vi "test - Convert config array - I8 - 1.vi"(8 "error in (no error)":errorcluster, 11 "TestCase in":refnum<class "Create New Assert Tester.lvclass">) -> (0 "error out":errorcluster, 3 "TestCase out":refnum<class "Create New Assert Tester.lvclass">)   [LabVIEW 2016, in "Create New Assert Tester.lvclass"]
uses:
  Create New Assert Tester.lvclass
  Plugins/Utility/Assert Build Configuration.ctl
  Core/Assert API Components/Failure Actions.ctl
  <vilib>/Utility/Data Type/Type Definitions/Data Type.ctl
  Plugins/Utility/Assert Scripting Configuration.ctl
  <vilib>/addons/_JKI Toolkits/VI Tester/TestCase.llb/TestCase.lvclass
  <vilib>/Utility/Data Type/NI_Data Type.lvlib
  Core/Assert API Components/Assert API Components.lvlib
  C:/Program Files (x86)/National Instruments/LabVIEW 2016/vi.lib/addons/_JKI Toolkits/VI Tester/TestCase.llb/TestCase.lvclass
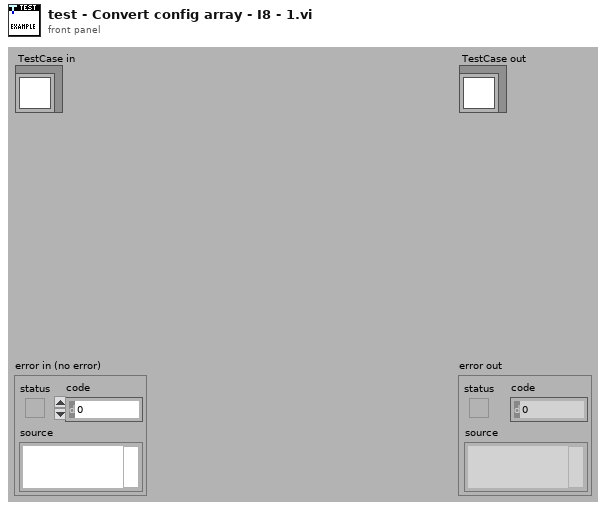
[diagram p1: front panel]
types:
  T1 = typedef "Assert Build Configuration.ctl" = cluster{"Assert Name":string, "Operation":string, "Comparison Value 1":string, "Comparison Value 2":string, "Comment":string, "Default Failure Action":T2, "Description":string, "Operation Display":string, "Active":bool, "Data Type":T3}
  T2 = typedef "Assert API Components.lvlib/Failure Actions.ctl" = enum16{"None", "Log To File", "Pause Execution", "Abort Execution"}
  T3 = typedef "NI_Data Type.lvlib/Data Type.ctl" = enum8{"Invalid Type", "Void", "I8", "I16", "I32", "I64", "U8", "U16", "U32", "U64", "Single Float", "Double Float", "Extended Float", "Single Complex", "Double Complex", "Extended Complex", "Enum U8", "Enum U16", "Enum U32", "Enum U64", "Single Float With Unit", "Double Float With Unit", "Extended Float With Unit", "Single Complex with Unit", "Double Complex with Unit", "Extended Complex with Unit", "Boolean", "String", "Path", "Picture", "Tag", "Array", "Cluster", "Variant", "LV Variant", "Waveform", "Timestamp", "Digital Waveform", "Digital Data", "ExpressData", "Refnum", "External Data", "VI", "Poly VI", "LabVIEW Class Instance", "Fixed Point"}
  T4 = enum16{"None", "Log To File", "Pause Execution", "Abort Execution"}
  T5 = typedef "Assert Scripting Configuration.ctl" = cluster{"Assert Name":string, "Comment":string, "Numeric Operation":string, "Type":T3, "String Operation":string, "DBL Comparison Value 1":dbl, "DBL Comparison Value 2":dbl, "I32 Comparison Value 1":i32, "I32 Comparison Value 2":i32, "Creator":string, "Creation Timestamp":timestamp, "String Comparison Value":string, "Description":string, "Default Failure Action":enum16{"None", "Log To File", "Pause Execution", "Abort Execution"}, "Boolean Comparison Value":bool, "I8 Comparison Value 1":i8, "I8 Comparison Value 2":i8, "I16 Comparison Value 1":i16, "I16 Comparison Value 2":i16, "I64 Comparison Value 1":i64, "I64 Comparison Value 2":i64, "U8 Comparison Value 1":u8, "U8 Comparison Value 2":u8, "U16 Comparison Value 1":u16, "U16 Comparison Value 2":u16, "U32 Comparison Value 1":u32, "U32 Comparison Value 2":u32, "U64 Comparison Value 1":u64, "U64 Comparison Value 2":u64, "EXT Comparison Value 1":ext, "EXT Comparison Value 2":ext, "SGL Comparison Value 1":sgl, "SGL Comparison Value 2":sgl}
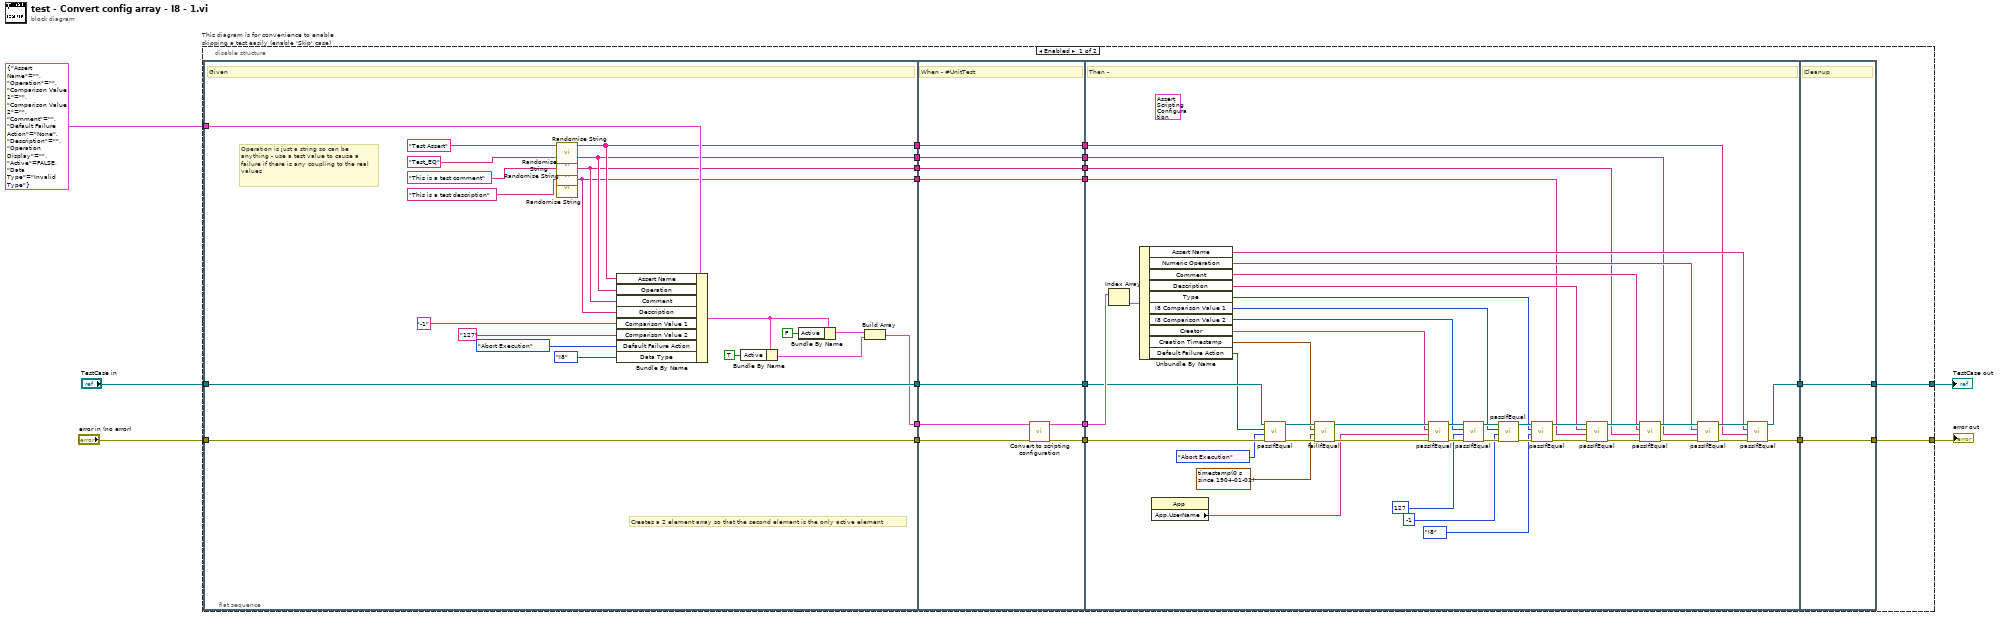
[diagram p0: block diagram]
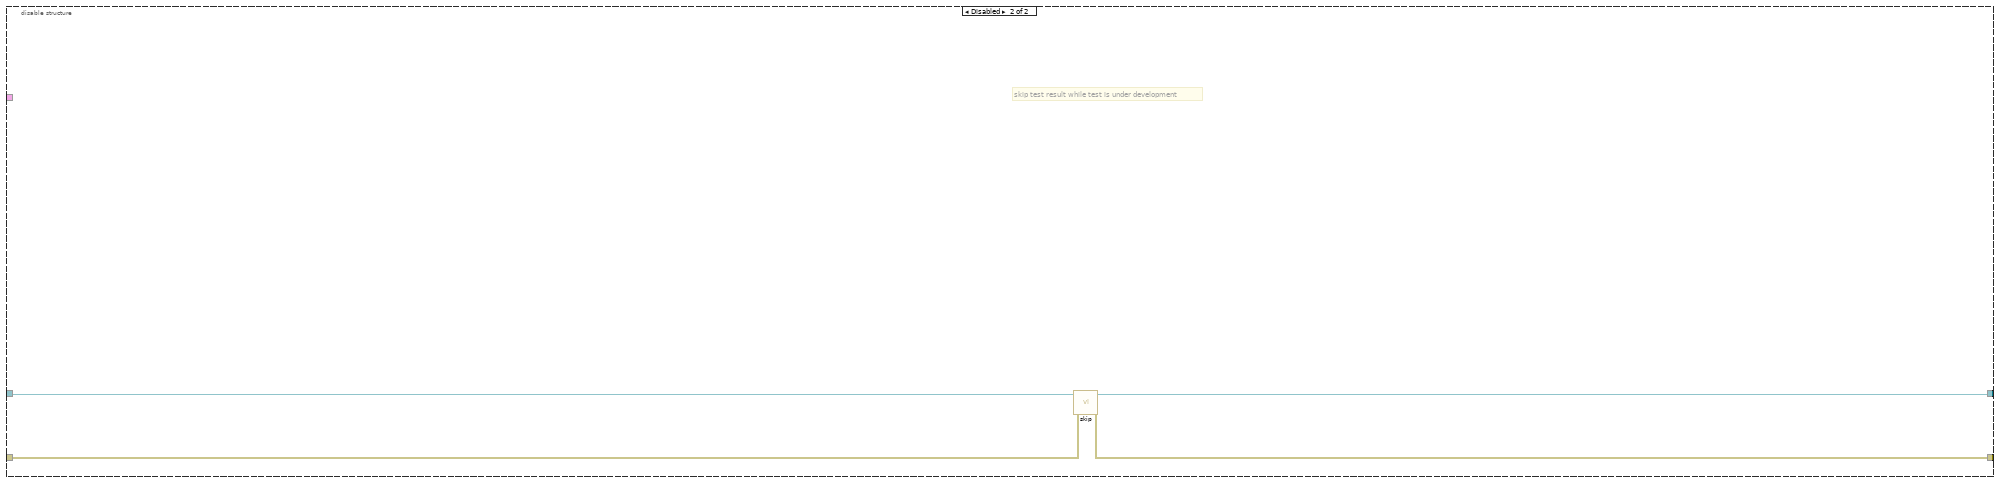
[diagram p2: hidden frame]
diagram:
  n1 = disable-structure "This diagram is for convenience to enable skipping a test easily (enable 'Skip' case)" shown="Enabled" {
    disable-tunnel: "TestCase in" -> [w20 w106]
    disable-tunnel: [w17 w104] -> w2
    disable-tunnel: [w18 w105] -> w4
    disable-tunnel: "error in (no error)" -> [w19 w103]
    disable-tunnel: T1 {"Assert Name"="", "Operation"="", "Comparison Value 1"="", "Comparison Value 2"="", "Comment"="", "Default Failure Action"=enum."None", "Description"="", "Operation Display"="", "Active"=FALSE, "Data Type"=enum."Invalid Type"} ("Assert Build Configuration") -> [w15 _]
    frame Enabled {
      n2 = flat-sequence {
        tunnel: w19 -> [w46]
        tunnel: w20 -> [w47]
        tunnel: [w47] -> w26
        tunnel: [w46] -> w25
        tunnel: w15 -> [w45]
        tunnel: [w40] -> w14
        tunnel: [w30] -> w12
        tunnel: [w29] -> w10
        tunnel: [w28] -> w8
        tunnel: [w27] -> w6
        tunnel: [w56] -> w24
        tunnel: [w54] -> w23
        tunnel: w26 -> [w56]
        tunnel: w25 -> [w55]
        tunnel: [w53] -> w16
        tunnel: w14 -> [w52]
        tunnel: [w51] -> w13
        tunnel: w12 -> [w51]
        tunnel: [w50] -> w11
        tunnel: w10 -> [w50]
        tunnel: [w49] -> w9
        tunnel: w8 -> [w49]
        tunnel: [w48] -> w7
        tunnel: w6 -> [w48]
        tunnel: [w62] -> w22
        tunnel: [w64] -> w21
        tunnel: w24 -> [w95]
        tunnel: w23 -> [w100]
        tunnel: w16 -> [w98]
        tunnel: w13 -> [w57]
        tunnel: w11 -> [w58]
        tunnel: w9 -> [w59]
        tunnel: w7 -> [w60]
        tunnel: [w101] -> w18
        tunnel: [w102] -> w17
        tunnel: w22 -> [w102]
        tunnel: w21 -> [w101]
        frame #0 {
          # "Creates a 2 element array so that the second element is the only active element"
          # "Operation is just a string so can be anything - use a test value to cause a failure if there is any coupling to the real values"
          # "Given"
          n3 = call "Randomise String.vi"("String in"="Test Assert" ("Assert Name")) -> ("String out"=w30:string)  [unwired: 10 in]
          n4 = call "Randomise String.vi"("String in"="Test_EQ" ("Operation")) -> ("String out"=w29:string)  [unwired: 10 in]
          n5 = call "Randomise String.vi"("String in"="This is a test comment" ("Comment")) -> ("String out"=w28:string)  [unwired: 10 in]
          n6 = call "Randomise String.vi"("String in"="This is a test description" ("Comment")) -> ("String out"=w27:string)  [unwired: 10 in]
          n7 = Bundle By Name(cluster=w45, "Assert Name"=w30, "Operation"=w29, "Comment"=w28, "Description"=w27, "Comparison Value 1"="-1" ("Comparison Value (Low)"), "Comparison Value 2"="127" ("Comparison Value (High)"), "Default Failure Action"=Failure_Actions."Abort Execution", "Data Type"=Data_Type."I8") -> (w37:T1)
          n8 = Bundle By Name(cluster=w37, "Active"=TRUE) -> (w35:T1)
          n9 = Bundle By Name(cluster=w37, "Active"=FALSE) -> (w39:T1)
          n10 = Build Array(w39, w35) -> (w40:T1[])
        }
        frame #1 {
          # "When - #UnitTest"
          n11 = call "Convert to scripting configuration.vi"("error in (no error)"=w55, "Multiple Assert Configuration"=w52) -> ("error out"=w54:errorcluster, "Array"=w53:T5[])  [unwired: 7 in, 1 out]
        }
        frame #2 {
          (unwired) T5 {"Assert Name"="", "Comment"="", "Numeric Operation"="", "Type"=enum."Invalid Type", "String Operation"="", "DBL Comparison Value 1"=0.0, "DBL Comparison Value 2"=0.0, "I32 Comparison Value 1"=0, "I32 Comparison Value 2"=0, "Creator"="", "Creation Timestamp"=timestamp(0 s since 1904-01-01), "String Comparison Value"="", "Description"="", "Default Failure Action"=enum."None", "Boolean Comparison Value"=FALSE, "I8 Comparison Value 1"=0, "I8 Comparison Value 2"=0, "I16 Comparison Value 1"=0, "I16 Comparison Value 2"=0, "I64 Comparison Value 1"=0, "I64 Comparison Value 2"=0, "U8 Comparison Value 1"=0, "U8 Comparison Value 2"=0, "U16 Comparison Value 1"=0, "U16 Comparison Value 2"=0, "U32 Comparison Value 1"=0, "U32 Comparison Value 2"=0, "U64 Comparison Value 1"=0, "U64 Comparison Value 2"=0, "EXT Comparison Value 1"=0.0, "EXT Comparison Value 2"=0.0, "SGL Comparison Value 1"=0.0, "SGL Comparison Value 2"=0.0} ("Assert Scripting Configuration")
          # "Then -"
          n12 = Index Array(array=w98) -> (element=w97:T5)  [unwired: 1 in]
          n13 = Unbundle By Name(w97) -> ("Assert Name"=w61:string, "Numeric Operation"=w72:string, "Comment"=w73:string, "Description"=w74:string, "Type"=w75:T3, "I8 Comparison Value 1"=w82:i8, "I8 Comparison Value 2"=w83:i8, "Creator"=w84:string, "Creation Timestamp"=w70:timestamp, "Default Failure Action"=w93:T4)
          n14 = property class="App"() -> ("App.UserName"=w68:string)  [unwired: 2 in, 2 out]
          n15 = call-dynamic "passIfEqual.vi"("error in (no error)"=w100, "y"=T4."Abort Execution" ("Default Failure Action"), "x"=w93, "TestCase in"=w95) -> ("error out"=w96:errorcluster, "TestCase out"=w94:refnum<class "Create New Assert Tester.lvclass">)  [unwired: 6 in]
          n16 = call-dynamic "failIfEqual.vi"("error in (no error)"=w96, "y"=timestamp(0 s since 1904-01-01) ("Creation Timestamp"), "x"=w70, "TestCase in"=w94) -> ("error out"=w99:errorcluster, "TestCase out"=w89:refnum<class "Create New Assert Tester.lvclass">)  [unwired: 6 in]
          n17 = call-dynamic "passIfEqual.vi"("error in (no error)"=w99, "y"=w68, "x"=w84, "TestCase in"=w89) -> ("error out"=w90:errorcluster, "TestCase out"=w88:refnum<class "Create New Assert Tester.lvclass">)  [unwired: 6 in]
          n18 = call-dynamic "passIfEqual.vi"("error in (no error)"=w90, "y"=i8 127 ("I8 Comparison Value 2"), "x"=w83, "TestCase in"=w88) -> ("error out"=w91:errorcluster, "TestCase out"=w86:refnum<class "Create New Assert Tester.lvclass">)  [unwired: 6 in]
          n19 = call-dynamic "passIfEqual.vi"("error in (no error)"=w91, "y"=i8 -1 ("I8 Comparison Value 1"), "x"=w82, "TestCase in"=w86) -> ("error out"=w87:errorcluster, "TestCase out"=w80:refnum<class "Create New Assert Tester.lvclass">)  [unwired: 6 in]
          n20 = call-dynamic "passIfEqual.vi"("error in (no error)"=w87, "y"=Data_Type."I8" ("Data Type"), "x"=w75, "TestCase in"=w80) -> ("error out"=w81:errorcluster, "TestCase out"=w79:refnum<class "Create New Assert Tester.lvclass">)  [unwired: 6 in]
          n21 = call-dynamic "passIfEqual.vi"("error in (no error)"=w81, "y"=w60, "x"=w74, "TestCase in"=w79) -> ("error out"=w85:errorcluster, "TestCase out"=w77:refnum<class "Create New Assert Tester.lvclass">)  [unwired: 6 in]
          n22 = call-dynamic "passIfEqual.vi"("error in (no error)"=w85, "y"=w59, "x"=w73, "TestCase in"=w77) -> ("error out"=w78:errorcluster, "TestCase out"=w76:refnum<class "Create New Assert Tester.lvclass">)  [unwired: 6 in]
          n23 = call-dynamic "passIfEqual.vi"("error in (no error)"=w78, "y"=w58, "x"=w72, "TestCase in"=w76) -> ("error out"=w92:errorcluster, "TestCase out"=w63:refnum<class "Create New Assert Tester.lvclass">)  [unwired: 6 in]
          n24 = call-dynamic "passIfEqual.vi"("error in (no error)"=w92, "y"=w57, "x"=w61, "TestCase in"=w63) -> ("error out"=w64:errorcluster, "TestCase out"=w62:refnum<class "Create New Assert Tester.lvclass">)  [unwired: 6 in]
        }
        frame #3 {
          # "Cleanup"
        }
      }
    }
    frame Disabled {
      # "skip test result while test is under development"
      n25 = call <vilib>:"skip.vi"("error in (no error)"=w103, "TestCase in"=w106) -> ("error out"=w105:errorcluster, "TestCase out"=w104:refnum<class "Create New Assert Tester.lvclass">)  [unwired: 8 in]
    }
  }
  "error out" <- w4
  "TestCase out" <- w2
